vi "RichToFlatnixnet_grpc_DbGetPropertyResponse.vi"(5 "OutputClusterType":T1, 11 "InputCluster":T5) -> (3 "OutputCluster":T1)   [LabVIEW 2025, in "xnet-grpc_client.lvlib"]
uses:
  nixnet_grpc_DbGetPropertyResponse.ctl
  nixnet_grpc_DbGetPropertyResponse_property_value/nixnet_grpc_DbGetPropertyResponse_property_value.lvclass
  nixnet_grpc_DbGetPropertyResponse_Flat.ctl
  nixnet_grpc_U32Array_Flat.ctl
  nidevice_grpc_Session_Flat.ctl
  nixnet_grpc_DbRefArray_Flat.ctl
  xnet-grpc_client.lvlib
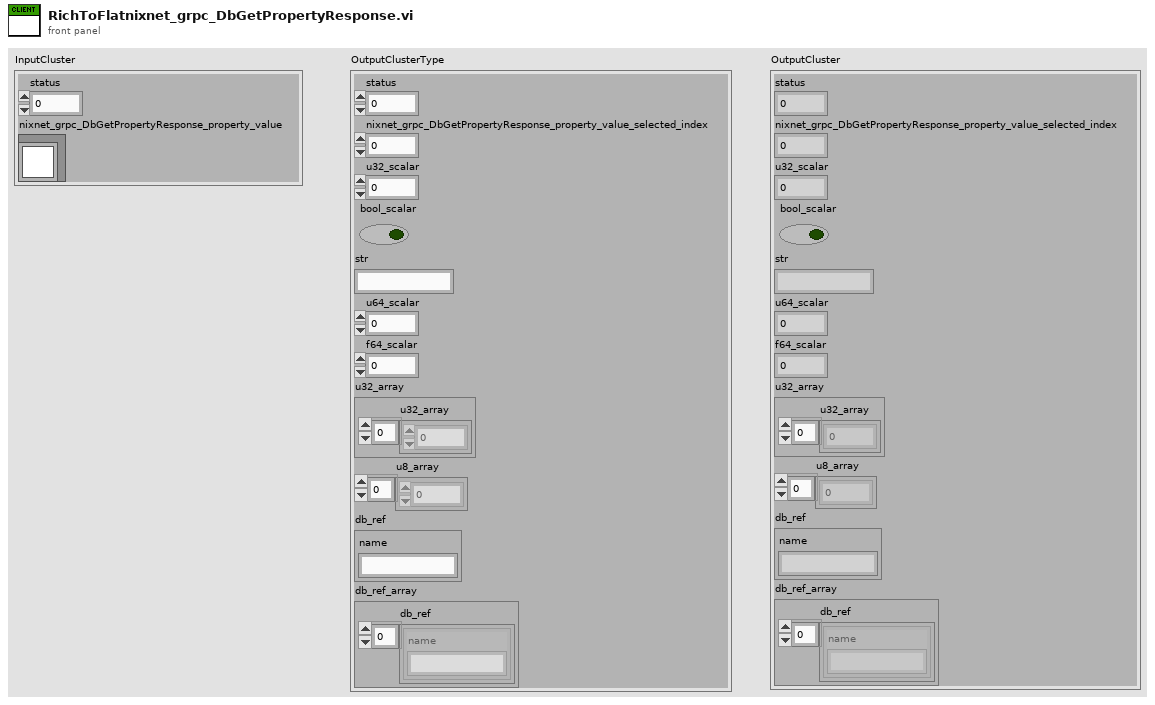
[diagram p1: front panel]
types:
  T1 = typedef "xnet-grpc_client.lvlib/nixnet_grpc_DbGetPropertyResponse_Flat.ctl" = cluster{"status":i32, "nixnet_grpc_DbGetPropertyResponse_property_value_selected_index":i32, "u32_scalar":u32, "bool_scalar":bool, "str":string, "u64_scalar":u64, "f64_scalar":dbl, "u32_array":T2, "u8_array":u8[], "db_ref":T3, "db_ref_array":T4}
  T2 = typedef "xnet-grpc_client.lvlib/nixnet_grpc_U32Array_Flat.ctl" = cluster{"u32_array":u32[]}
  T3 = typedef "xnet-grpc_client.lvlib/nidevice_grpc_Session_Flat.ctl" = cluster{"name":string}
  T4 = typedef "xnet-grpc_client.lvlib/nixnet_grpc_DbRefArray_Flat.ctl" = cluster{"db_ref":T3[]}
  T5 = typedef "xnet-grpc_client.lvlib/nixnet_grpc_DbGetPropertyResponse.ctl" = cluster{"status":i32, "nixnet_grpc_DbGetPropertyResponse_property_value":refnum<class "nixnet_grpc_DbGetPropertyResponse_property_value.lvclass">}
  T6 = typedef "xnet-grpc_client.lvlib/nixnet_grpc_U32Array.ctl" = cluster{"u32_array":u32[]}
  T7 = typedef "xnet-grpc_client.lvlib/nidevice_grpc_Session.ctl" = cluster{"name":string}
  T8 = typedef "xnet-grpc_client.lvlib/nixnet_grpc_DbRefArray.ctl" = cluster{"db_ref":T7[]}
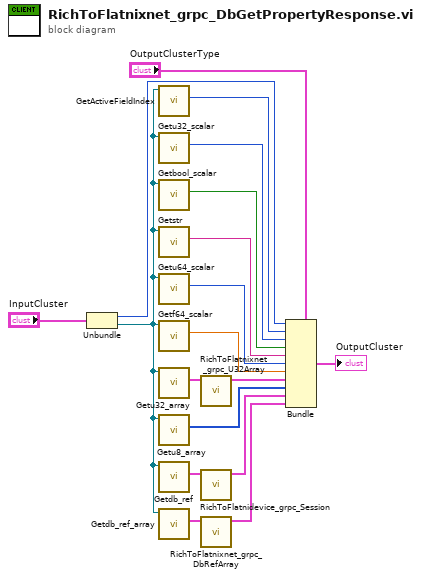
[diagram p0: block diagram]
diagram:
  n1 = Unbundle "Unbundle"("InputCluster") -> ("status"=w15:i32, "nixnet_grpc_DbGetPropertyResponse_property_value"=w14:refnum<class "nixnet_grpc_DbGetPropertyResponse_property_value.lvclass">)
  n2 = call "GetActiveFieldIndex.vi"("OneOfTemplate in"=w14) -> ("Active Field Index"=w13:i32)  [unwired: 8 in, 2 out]
  n3 = call "Getu32_scalar.vi"("OneOfTemplate in"=w14) -> ("Get_Val"=w12:u32)  [unwired: 8 in, 2 out]
  n4 = call "Getbool_scalar.vi"("OneOfTemplate in"=w14) -> ("Get_Val"=w11:bool)  [unwired: 8 in, 2 out]
  n5 = call "Getstr.vi"("OneOfTemplate in"=w14) -> ("Get_Val"=w10:string)  [unwired: 8 in, 2 out]
  n6 = call "Getu64_scalar.vi"("OneOfTemplate in"=w14) -> ("Get_Val"=w9:u64)  [unwired: 8 in, 2 out]
  n7 = call "Getf64_scalar.vi"("OneOfTemplate in"=w14) -> ("Get_Val"=w8:dbl)  [unwired: 8 in, 2 out]
  n8 = call "Getu32_array.vi"("OneOfTemplate in"=w14) -> ("Get_Val"=w7:T6)  [unwired: 8 in, 2 out]
  n9 = call "Getu8_array.vi"("OneOfTemplate in"=w14) -> ("Get_Val"=w5:u8[])  [unwired: 8 in, 2 out]
  n10 = call "Getdb_ref.vi"("OneOfTemplate in"=w14) -> ("Get_Val"=w4:T7)  [unwired: 8 in, 2 out]
  n11 = call "Getdb_ref_array.vi"("OneOfTemplate in"=w14) -> ("Get_Val"=w2:T8)  [unwired: 8 in, 2 out]
  n12 = call "RichToFlatnixnet_grpc_U32Array.vi"("InputCluster"=w7) -> ("OutputCluster"=w6:T2)  [unwired: 10 in]
  n13 = call "RichToFlatnidevice_grpc_Session.vi"("InputCluster"=w4) -> ("OutputCluster"=w3:T3)  [unwired: 10 in]
  n14 = call "RichToFlatnixnet_grpc_DbRefArray.vi"("InputCluster"=w2) -> ("OutputCluster"=w1:T4)  [unwired: 10 in]
  n15 = Bundle "Bundle"(cluster="OutputClusterType", "status"=w15, "nixnet_grpc_DbGetPropertyResponse_property_value_selected_index"=w13, "u32_scalar"=w12, "bool_scalar"=w11, "str"=w10, "u64_scalar"=w9, "f64_scalar"=w8, "u32_array"=w6, "u8_array"=w5, "db_ref"=w3, "db_ref_array"=w1) -> (→"OutputCluster":T1)
